vi "OAT Calculate Orbit Precession Direction.vi"(4 "revolutions":dbl format="%.2f", 6 "actual samples/rev":dbl format="%.2f", 7 "tach duty":i32=1, 8 "error in (no error)":errorcluster, 9 "max axis value":dbl format="%.2f", 10 "shaft rotating direction":u16, 11 "XY plot data in":cluster{dbl[], dbl[]}[](array[cluster]) {"?" format="%.2f"; "?" format="%.2f"}) -> (0 "error out":errorcluster, 1 "max value":dbl, 2 "orbit precession direction":u16(ring) items=["forward", "backward"], 3 "XY plot data out":cluster{dbl[], dbl[]}[](array[cluster]) {"?" format="%.2f"; "?" format="%.2f"})   [LabVIEW 2017]
uses:
  <vilib>/Analysis/1siggen.llb/Ramp Pattern by Samples.vi
  <vilib>/Analysis/NI_AALPro.lvlib
  <vilib>/Analysis/NI_AALBase.lvlib
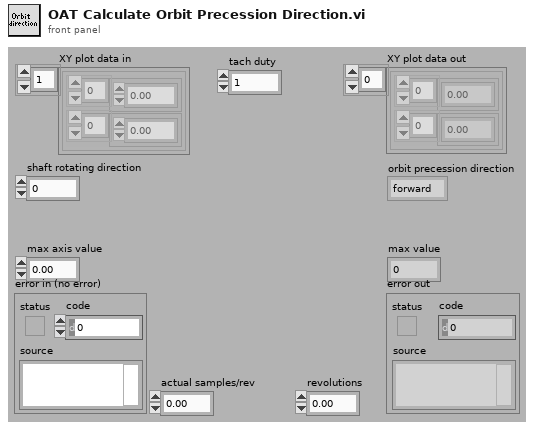
[diagram p1: front panel]
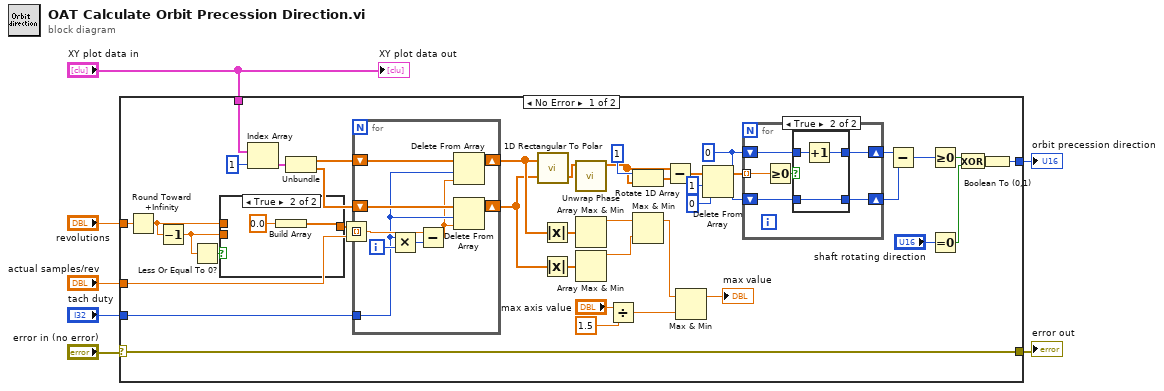
[diagram p0: block diagram]
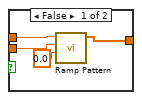
[diagram p2: hidden frame]
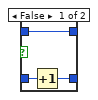
[diagram p3: hidden frame]
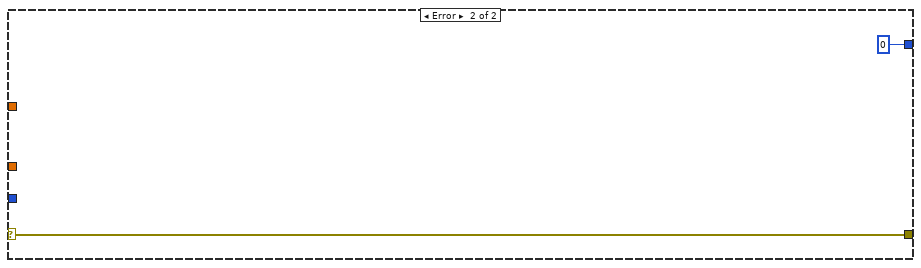
[diagram p4: hidden frame]
diagram:
  n1 = case shown="No Error" "error in (no error)" {
    selector: "error in (no error)" -> [w8 w78]
    tunnel: [w49 i16 0] -> w7
    tunnel: "XY plot data in" -> [w44 _]
    tunnel: "revolutions" -> [w22 _]
    tunnel: "tach duty" -> [w21 _]
    tunnel: "actual samples/rev" -> [w19 _]
    tunnel: [w8 w78] -> w1
    frame No Error {
      w24 = 0
      n2 = Round Toward +Infinity(x=w22) -> (ceil(x): smallest int >= x=w11:dbl)
      n3 = Decrement(x=w11) -> (x-1=w9:dbl)
      n4 = Less Or Equal To 0?(x=w9) -> (x <= 0?=w10:bool)
      n5 = case shown="True" w10 {
        tunnel: w11 -> [w52 _]
        tunnel: w9 -> [w51 _]
        tunnel: [w50 w55] -> w18
        frame False {
          n6 = call-poly <vilib>:"Ramp Pattern.vi"("start"=0.0, "end"=w51, "samples"=w52) -> ("Ramp Pattern"=w50:dbl[])  [unwired: 7 in, 1 out]
        }
        frame True {
          n7 = Build Array(0.0 ("element")) -> (w55:dbl[])
        }
      }
      n8 = Index Array(array=w44, index=1) -> (element=w33:cluster{dbl[], dbl[]})
      n9 = Unbundle(w33) -> (w20:dbl[], w16:dbl[])
      n10 = Multiply(x=w18, y=w19) -> (x*y=w17:dbl[])
      n11 = for {
        tunnel: w21 -> [w57]
        shift-right: [w63] -> w15
        shift-left: w20 -> [w64]
        tunnel: w17 -> [w62] mode=indexing
        shift-right: [w58] -> w14
        shift-left: w16 -> [w59]
        i -> [w61]
        n12 = Multiply(x=w57, y=w61) -> (x*y=w60:i32)
        n13 = Subtract(x=w62, y=w60) -> (x-y=w56:dbl)
        n14 = Delete From Array(array=w64, length=w57, index=w56) -> (array with subset deleted=w63:dbl[])  [unwired: 1 out]
        n15 = Delete From Array(array=w59, length=w57, index=w56) -> (array with subset deleted=w58:dbl[])  [unwired: 1 out]
      }
      n16 = call <vilib>:"1D Rectangular To Polar.vi"("X"=w15, "Y"=w14) -> ("Phase"=w25:dbl[])  [unwired: 2 out]
      n17 = Absolute Value(x=w15) -> (abs(x)=w42:dbl[])
      n18 = Absolute Value(x=w14) -> (abs(x)=w41:dbl[])
      n19 = call <vilib>:"Unwrap Phase.vi"("Phase"=w25) -> ("Unwrapped Phase"=w27:dbl[])  [unwired: 9 in, 1 out]
      n20 = Array Max & Min(array=w42) -> (max value=w40:dbl)  [unwired: 3 out]
      n21 = Array Max & Min(array=w41) -> (max value=w39:dbl)  [unwired: 3 out]
      n22 = Divide(x="max axis value", y=1.5) -> (x/y=w36:dbl)
      n23 = Rotate 1D Array(1:w27, 2:1 ("n")) -> (0:w29:dbl[])
      n24 = Max & Min(x=w40, y=w39) -> (max(x,y)=w35:dbl)  [unwired: 1 out]
      n25 = Subtract(x=w27, y=w29) -> (x-y=w30:dbl[])
      n26 = Max & Min(x=w35, y=w36) -> (max(x,y)=→"max value":dbl)  [unwired: 1 out]
      n27 = Delete From Array(array=w30, length=1, index=0) -> (array with subset deleted=w26:dbl[])  [unwired: 1 out]
      n28 = for {
        tunnel: w26 -> [w70] mode=indexing
        shift-right: [w66] -> w13
        shift-left: w24 -> [w68]
        shift-right: [w65] -> w12
        shift-left: w24 -> [w67]
        n29 = Greater Or Equal To 0?(x=w70) -> (x >= 0?=w69:bool)
        n30 = case shown="True" w69 {
          tunnel: w68 -> [w73 w76]
          tunnel: w67 -> [w72 w74]
          tunnel: [w73 w75] -> w66
          tunnel: [w71 w74] -> w65
          frame False {
            n31 = Increment(x=w72) -> (x+1=w71:i32)
          }
          frame True {
            n32 = Increment(x=w76) -> (x+1=w75:i32)
          }
        }
      }
      n33 = Subtract(x=w13, y=w12) -> (x-y=w43:i32)
      n34 = Greater Or Equal To 0?(x=w43) -> (x >= 0?=w46:bool)
      n35 = Equal To 0?(x="shaft rotating direction") -> (x = 0?=w47:bool)
      n36 = Exclusive Or(1:w47, 2:w46) -> (0:w48:bool)
      n37 = Boolean To (0,1)(Boolean=w48) -> (0, 1=w49:i16)
    }
    frame Error {
    }
  }
  "orbit precession direction" <- w7
  "error out" <- w1
  "XY plot data out" <- "XY plot data in"
